vi "pressure and IK2 2016.vi"(3 "Ft. of SS":dbl=45.0 format="%.2f", 4 "flow":dbl=10.0 format="%.2f") -> (0 "Corrected Headloss":dbl=60.584999999999994 format="%.2f", 1 "IK":dbl=0.16505735743170755 format="%.4f")   [LabVIEW 2016]
uses:
  Kpro Globals.vi
panel:
  out "Total Pressure":dbl=61.8 format="%.2f"
  out "Current Depth":sgl=30.0 format="%.2f"
  out "Depth to Water Table":dbl=27.0 format="%.2f"
  out "depth out":dbl=27.0 format="%.2f"
  out "Head Loss":dbl=1.2149999999999999 format="%.2f"
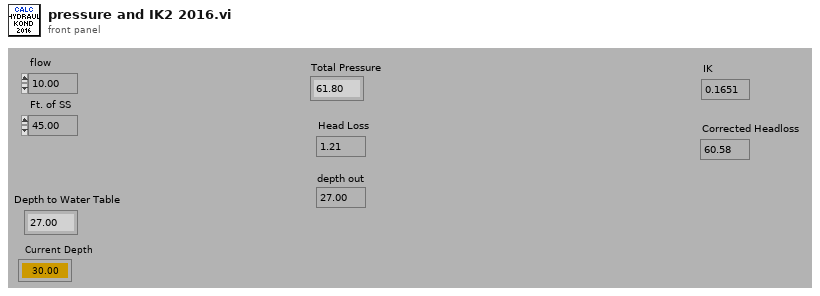
[diagram p1: front panel]
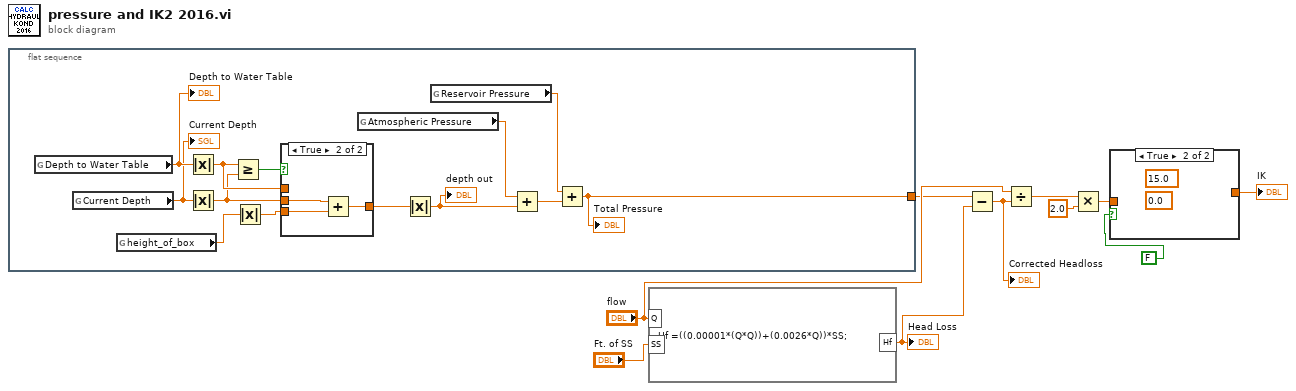
[diagram p0: block diagram]
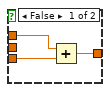
[diagram p2: hidden frame]
diagram:
  n1 = flat-sequence {
    tunnel: [w20] -> w6
    frame #0 {
      n2 = global read "Kpro Globals.vi" "Depth to Water Table"() -> (w19:dbl)
      "Depth to Water Table" <- w19
      n3 = global read "Kpro Globals.vi" "Current Depth"() -> (w15:sgl)
      "Current Depth" <- w15
      n4 = global read "Kpro Globals.vi" "height_of_box"() -> (w14:dbl)
      n5 = Absolute Value(x=w19) -> (abs(x)=w12:dbl)
      n6 = Absolute Value(x=w15) -> (abs(x)=w11:sgl)
      n7 = Greater Or Equal?(x=w12, y=w11) -> (x >= y?=w23:bool)
      n8 = Absolute Value(x=w14) -> (abs(x)=w13:dbl)
      n9 = case shown="True" w23 {
        tunnel: [w26 w29] -> w17
        tunnel: w13 -> [w25 w28]
        tunnel: w11 -> [_ w27]
        tunnel: w12 -> [w24 _]
        frame False {
          n10 = Add(x=w24, y=w25) -> (x+y=w26:dbl)
        }
        frame True {
          n11 = Add(x=w27, y=w28) -> (x+y=w29:dbl)
        }
      }
      n12 = global read "Kpro Globals.vi" "Atmospheric Pressure"() -> (w22:dbl)
      n13 = Absolute Value(x=w17) -> (abs(x)=w18:dbl)
      "depth out" <- w18
      n14 = global read "Kpro Globals.vi" "Reservoir Pressure"() -> (w16:dbl)
      n15 = Add(x=w22, y=w18) -> (x+y=w21:dbl)
      n16 = Add(x=w16, y=w21) -> (x+y=w20:dbl)
      "Total Pressure" <- w20
    }
  }
  n17 = formula code="Hf =((0.00001*(Q*Q))+(0.0026*Q))*SS;"("Q"="flow", "SS"="Ft. of SS") -> ("Hf"=w5:dbl)
  "Head Loss" <- w5
  n18 = Subtract(x=w6, y=w5) -> (x-y=w4:dbl)
  "Corrected Headloss" <- w4
  n19 = Divide(x="flow", y=w4) -> (x/y=w7:dbl)
  n20 = Multiply(x=w7, y=2.0) -> (x*y=w3:dbl)
  n21 = case shown="True" FALSE ("Simulate AD6B") {
    tunnel: [w30 _] -> w2
    tunnel: w3 -> [w30 _]
    frame False {
    }
    frame True {
      (unwired) 0.0 ("value_low")
      (unwired) 15.0 ("value_high")
    }
  }
  "IK" <- w2
